vi "LED-Set Text_Label.vi"() -> (0 "\"Set Text\" Label":string)   [LabVIEW 2010, in "LED Display.xctl"]
uses:
  LED Display.xctl
panel:
  in  "String":string="Set Text"
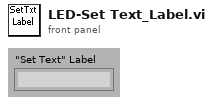
[diagram p1: front panel]
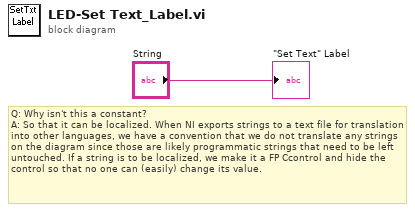
[diagram p0: block diagram]
diagram:
  # "Q: Why isn't this a constant?\nA: So that it can be localized. When NI exports strings to a text file for translation into other languages, we have a convention that we do not translate any strings on the diagram since those are likely programmatic strings that need to be left untouched. If a string is to be localized, we make it a FP Ccontrol and hide the control so that no one can (easily) change its value."
  "\"Set Text\" Label" <- "String"
